vi "SetJSONData.vi"(0 "reference in":refnum<class "String.lvclass">, 1 "VI Reference":refnum<vi>, 2 "Value":string, 5 "error in (no error)":errorcluster) -> (14 "reference out":refnum<class "String.lvclass">, 19 "error out":errorcluster)   [LabVIEW 2014, in "String.lvclass"]
uses:
  String.lvclass
  Object_class/Object.lvclass
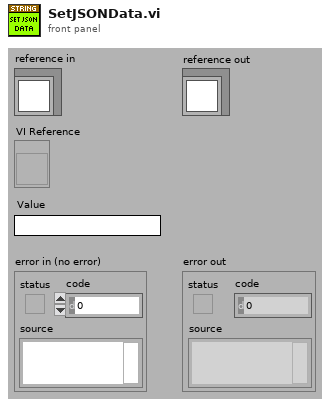
[diagram p1: front panel]
types:
  T1 = typedef "Object.lvclass/Attributes.ctl" = cluster{"UID":i32, "Type":string, "Coordinates":T2, "Reference":refnum<vi>}
  T2 = typedef "Object.lvclass/Coordinates.ctl" = cluster{"Left":i32, "Top":i32, "Height":u32, "Width":u32}
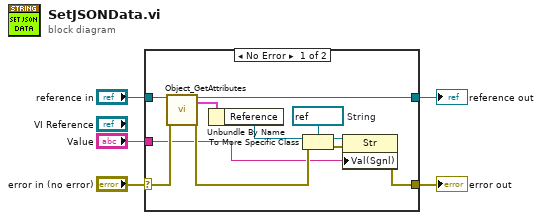
[diagram p0: block diagram]
diagram:
  n1 = case shown="No Error" "error in (no error)" {
    selector: "error in (no error)" -> [w16 w18]
    tunnel: [w15 w18] -> w4
    tunnel: [w10 w17] -> w2
    tunnel: "reference in" -> [w11 w17]
    tunnel: "Value" -> [w8 _]
    frame No Error {
      w6 = refnum<vi> refnum  # String
      n2 = call "Object_GetAttributes.vi"("reference in"=w11, "error in (no error)"=w16) -> ("reference out"=w10:refnum<class "String.lvclass">, "Data"=w12:T1, "error out"=w14:errorcluster)  [unwired: 14 in, 1 out]
      n3 = Unbundle By Name(w12) -> ("Reference"=w9:refnum<vi>)
      n4 = To More Specific Class(target class=w6, reference=w9, error in=w14) -> (specific class reference=w7:refnum<vi>, error out=w13:errorcluster)
      n5 = property class="Str"(reference=w7, error in=w13, "Val(Sgnl)"=w8) -> (error out=w15:errorcluster)  [unwired: 1 out]
    }
    frame Error {
    }
  }
  "error out" <- w4
  "reference out" <- w2
